vi "Add Message Buffer (BC).vi"(6 "MessageData (0x0000)":u16[](array[numeric]) format="%04x", 8 "error in":errorcluster, 9 "MessageBuffer configuration":T1={"bufferMaxEntries"=1, "bufferType"=0, "eventLogOnEmptyOrFull"=FALSE, "eventLogOnHalf"=FALSE} {"bufferType" items=["FIFO", "Circular"]}, 10 "name":string="CoreName", 11 "Bus Controllerl in":refnum<k24>) -> (0 "error out":errorcluster, 1 "ID out":i32, 2 "new messageBuffer":refnum<k24>, 3 "Bus Controller out":refnum<k24>)   [LabVIEW 2020, in "Ballard_1553_Hardware_ni.lvlib"]
uses:
  Ballard_1553_Hardware_ni.lvlib
  C:/Users/Administrator/Desktop/GIT/Ballard-MIL-STD-1553-Custom-Device/Source/System Explorer/SubVIs/Parse XML Ballard/1.2/BTIXML_SerDes.dll
  Ballard-MIL-STD-1553-Custom-Device/Source/System Explorer/SubVIs/Parse XML Ballard/1.2/BTIXML_SerDes.dll
  _typedefs/MessageBuffer_type.ctl
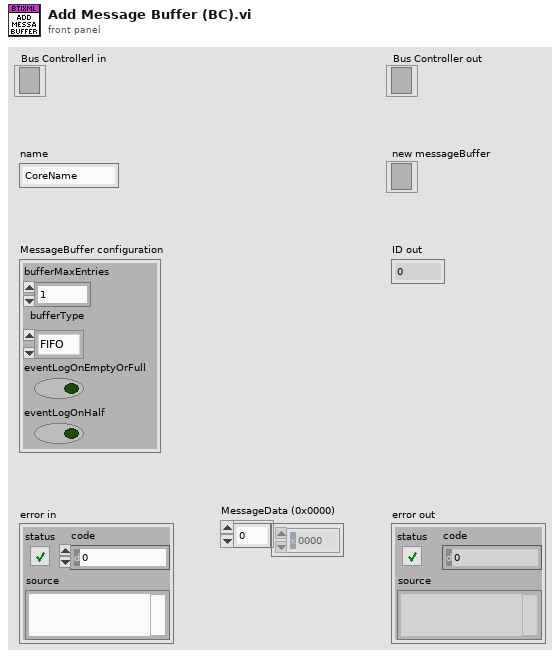
[diagram p1: front panel]
types:
  T1 = typedef "Ballard_1553_Hardware_ni.lvlib/MessageBuffer_type.ctl" = cluster{"bufferMaxEntries":i32, "bufferType":i32, "eventLogOnEmptyOrFull":bool, "eventLogOnHalf":bool}
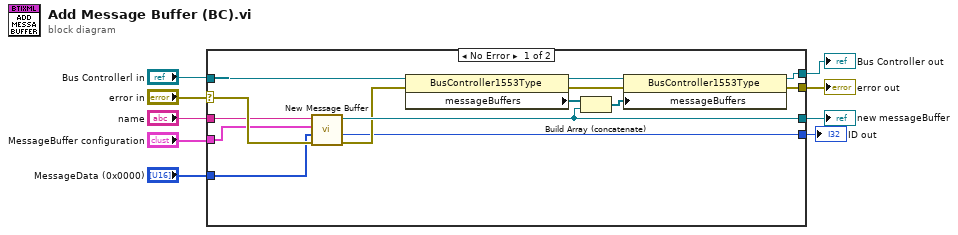
[diagram p0: block diagram]
diagram:
  n1 = case shown="No Error" "error in" {
    selector: "error in" -> [w15 w24]
    tunnel: [w21 w24] -> w9
    tunnel: [w22 w25] -> w8
    tunnel: "Bus Controllerl in" -> [w23 w25]
    tunnel: [w17 _] -> w5
    tunnel: [w13 _] -> w4
    tunnel: "name" -> [w12 _]
    tunnel: "MessageBuffer configuration" -> [w11 _]
    tunnel: "MessageData (0x0000)" -> [w10 _]
    frame No Error {
      n2 = call "New Message Buffer.vi"("error in"=w15, "MessageData (0x0000)"=w10, "MessageBuffer configuration"=w11, "name"=w12) -> ("error out"=w14:errorcluster, "ID out"=w13:i32, "new messageBuffer"=w17:refnum<k24>)  [unwired: 5 in]
      n3 = property class="BusController1553Type"(reference=w23, error in=w14) -> (reference out=w19:refnum<k24>, error out=w20:errorcluster, "messageBuffers"=w18:refnum<k24>[])
      n4 = Build Array (concatenate)(w18, w17) -> (w16:refnum<k24>[])
      n5 = property class="BusController1553Type"(reference=w19, error in=w20, "messageBuffers"=w16) -> (reference out=w22:refnum<k24>, error out=w21:errorcluster)
    }
    frame Error {
    }
  }
  "error out" <- w9
  "Bus Controller out" <- w8
  "new messageBuffer" <- w5
  "ID out" <- w4
